vi "Utilization Test.vi"() -> ()   [LabVIEW 2019]
uses:
  Asset External Calibration/Asset External Calibration.lvclass
  <vilib>/Skyline/AssetManagement/Start Utilization (All).vi
  <vilib>/Skyline/AssetManagement/Start Utilization (Single).vi
  Asset/Asset.lvclass
  <vilib>/Skyline/AssetManagement/NI SystemLink Asset Utilization.lvclass
  <vilib>/Skyline/Utilities/NI Skyline Utilities.lvlib
panel:
  in  "Number of assets":i32=10
  out "Assets":string[](array[string])
  out "Iteration":i32
  in  "stop":bool
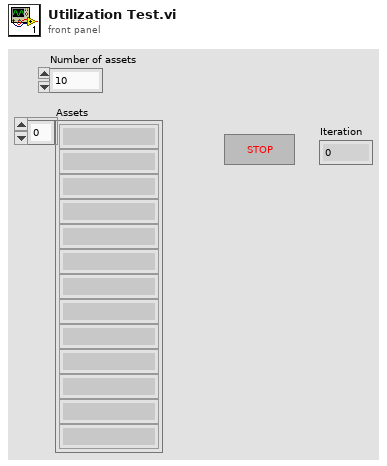
[diagram p1: front panel]
types:
  T1 = enum16{"BuiltInSystem", "PciPxi", "Usb", "Gpib", "Vxi", "Serial", "TcpIp", "cRio", "Scxi", "cDaq", "SwitchBlock", "Scc", "FireWire", "Accessory", "Can", "SwitchBlockDevice"}
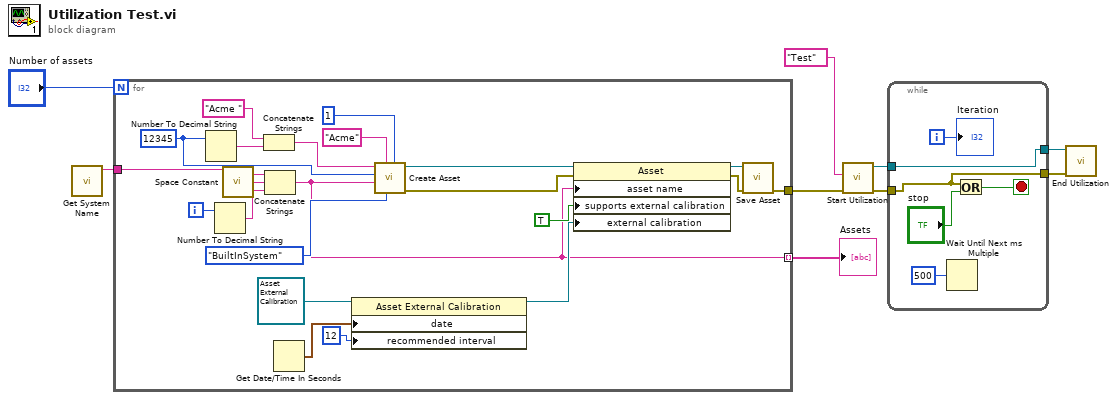
[diagram p0: block diagram]
diagram:
  n1 = call <vilib>:"Get System Name.vi"() -> ("system name"=w2:string)  [unwired: 11 in]
  n2 = for {
    N: "Number of assets" -> [_]
    tunnel: [w29] -> w5
    tunnel: w2 -> [w17]
    tunnel: [w10] -> w1 mode=indexing
    i -> [w16]
    w14 = u32 12345 ("Model Number")
    n3 = Number To Decimal String(number=w14) -> (decimal integer string=w12:string)  [unwired: 1 in]
    n4 = Number To Decimal String(number=w16) -> (decimal integer string=w15:string)  [unwired: 1 in]
    n5 = call <vilib>:"Space Constant.vi"() -> ("String"=w13:string)
    n6 = Concatenate Strings("Acme " ("Model Name"), w12) -> (w11:string)
    n7 = Concatenate Strings(w17, w13, w15) -> (w10:string)
    n8 = Get Date/Time In Seconds() -> (seconds since 1Jan1904=w19:timestamp)
    n9 = property class="Asset External Calibration"(reference=refnum<class "Asset External Calibration.lvclass"> refnum ("external calibration"), "date"=w19, "recommended interval"=u32 12) -> (reference out=w20:refnum<class "Asset External Calibration.lvclass">)  [unwired: 1 in, 1 out]
    n10 = call "Create Asset.vi"("Vendor Number"=u32 1, "Bus Type"=T1."BuiltInSystem", "Vendor Name"="Acme", "Serial Number"=w10, "Model Number"=w14, "Model Name"=w11) -> ("Error Out"=w27:errorcluster, "Asset"=w24:refnum<class "Asset.lvclass">)  [unwired: 4 in]
    n11 = property class="Asset"(reference=w24, error in=w27, "asset name"=w10, "supports external calibration"=TRUE, "external calibration"=w20) -> (reference out=w25:refnum<class "Asset.lvclass">, error out=w26:errorcluster)
    n12 = call "Save Asset.vi"("Error In"=w26, "Asset"=w25) -> ("Error Out"=w29:errorcluster)  [unwired: 9 in]
  }
  "Assets" <- w1
  n13 = call-poly <vilib>:"Start Utilization.vi"("error in (no error)"=w5, "utilization category"="Test") -> ("error out"=w8:errorcluster, "asset utilization"=w9:refnum<class "NI SystemLink Asset Utilization.lvclass">)  [unwired: 8 in]
  n14 = while {
    tunnel: [w36] -> w6
    tunnel: w9 -> [w36]
    tunnel: w8 -> [w35]
    tunnel: [w35] -> w7
    i -> [w32]
    stop <- w33 stop-if-true
    n15 = Wait Until Next ms Multiple(millisecond multiple=u32 500) -> ()  [unwired: 1 out]
    n16 = Or(x=w35, y="stop") -> (x .or. y?=w33:bool)
    "Iteration" <- w32
  }
  n17 = call <vilib>:"End Utilization.vi"("error in (no error)"=w7, "asset utilization"=w6) -> ()  [unwired: 9 in, 1 out]
